vi "Get factory trim.vi"(8 "error in (no error)":errorcluster, 11 "Accelerometer":T1) -> (0 "error out":errorcluster, 1 "Accel trim":dbl[](array[numeric]), 2 "Gyro trim":dbl[](array[numeric]), 3 "Accelerometer out":T1)   [LabVIEW 2013]
doc: "Use this template to build a VI to use as a subVI."
uses:
  AccelerometerSPI.ctl
  <vilib>/ni845x/ni845x.llb/ni845xControl.ctl
  <vilib>/ni845x/ni845x.llb/ni845xSpiConfiguration.ctl
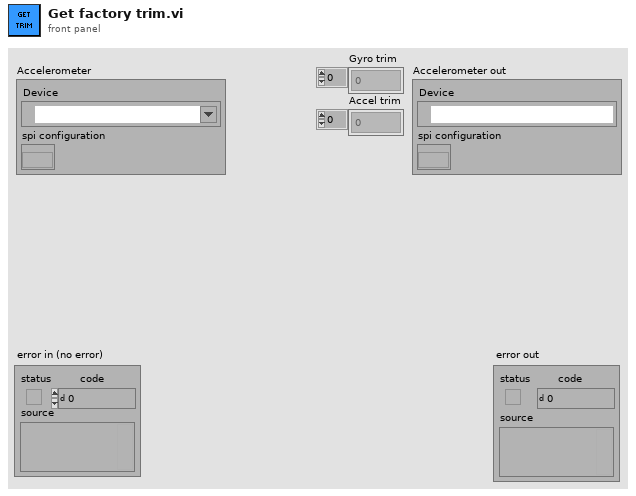
[diagram p1: front panel]
types:
  T1 = typedef "AccelerometerSPI.ctl" = cluster{"Device":T2, "spi configuration":T3}
  T2 = typedef "ni845xControl.ctl" = refnum<k21>
  T3 = typedef "ni845xSpiConfiguration.ctl" = refnum<k20>
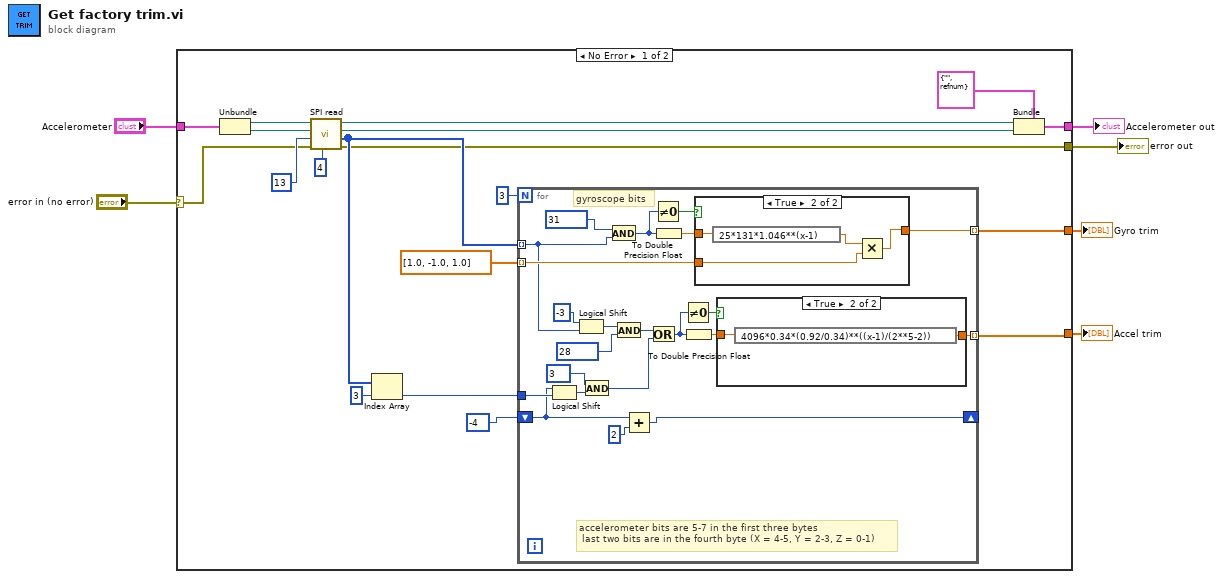
[diagram p0: block diagram]
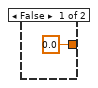
[diagram p2: hidden frame]
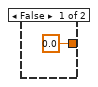
[diagram p3: hidden frame]
diagram:
  n1 = case shown="No Error" "error in (no error)" {
    selector: "error in (no error)" -> [w21 w57]
    tunnel: [w10 w57] -> w5
    tunnel: "Accelerometer" -> [w25 w56]
    tunnel: [w11 w56] -> w3
    tunnel: [w9 _] -> w2
    tunnel: [w8 _] -> w1
    frame No Error {
      n2 = Unbundle(w25) -> ("Device"=w24:T2, "spi configuration"=w23:T3)
      n3 = call "SPI read.vi"("Number of bytes"=4, "error in (no error)"=w21, "Address"=u8 13, "spi configuration in"=w23, "Device ref in"=w24) -> ("error out"=w10:errorcluster, "read data"=w17:u8[], "spi configuration out"=w13:T3, "Device ref out"=w14:T2)  [unwired: 3 in]
      n4 = Index Array(array=w17, index=3) -> (element=w15:u8)
      n5 = for {
        N: 3 -> [_]
        tunnel: w17 -> [w40] mode=indexing
        tunnel: dbl[] [1.0, -1.0, 1.0] ("read data") -> [w43] mode=indexing
        tunnel: [w42] -> w9 mode=indexing
        tunnel: w15 -> [w32]
        shift-right: [w27] -> _
        shift-left: i8 -4 ("Address") -> [w29]
        tunnel: [w33] -> w8 mode=indexing
        # "accelerometer bits are 5-7 in the first three bytes\n last two bits are in the fourth byte (X = 4-5, Y = 2-3, Z = 0-1)"
        # "gyroscope bits"
        n6 = Logical Shift(y=w29, x=w32) -> (x << y=w31:u8)
        n7 = Logical Shift(y=i16 -3, x=w40) -> (x << y=w39:u8)
        n8 = And(x=u8 3 ("Address"), y=w31) -> (x .and. y?=w26:u8)
        n9 = And(x=u8 31 ("Address"), y=w40) -> (x .and. y?=w45:u8)
        n10 = And(x=w39, y=u8 28 ("Address")) -> (x .and. y?=w37:u8)
        n11 = Add(x=w29, y=i8 2) -> (x+y=w27:i8)
        n12 = Or(x=w37, y=w26) -> (x .or. y?=w34:u8)
        n13 = Not Equal To 0?(x=w45) -> (x != 0?=w46:bool)
        n14 = To Double Precision Float(number=w45) -> (double precision float=w44:dbl)
        n15 = Not Equal To 0?(x=w34) -> (x != 0?=w35:bool)
        n16 = To Double Precision Float(number=w34) -> (double precision float=w36:dbl)
        n17 = case shown="True" w46 {
          tunnel: w44 -> [_ w55]
          tunnel: w43 -> [_ w53]
          tunnel: [0.0 w52] -> w42
          frame False {
          }
          frame True {
            n18 = expression code="25*131*1.046**(x-1)"(w55) -> (w54:dbl)
            n19 = Multiply(x=w54, y=w53) -> (x*y=w52:dbl)
          }
        }
        n20 = case shown="True" w35 {
          tunnel: w36 -> [_ w50]
          tunnel: [0.0 w49] -> w33
          frame False {
          }
          frame True {
            n21 = expression code="4096*0.34*(0.92/0.34)**((x-1)/(2**5-2))"(w50) -> (w49:dbl)
          }
        }
      }
      n22 = Bundle(cluster=T1 {"Device"="", "spi configuration"=refnum} ("Accelerometer"), "Device"=w14, "spi configuration"=w13) -> (w11:T1)
    }
    frame Error {
    }
  }
  "error out" <- w5
  "Accelerometer out" <- w3
  "Gyro trim" <- w2
  "Accel trim" <- w1
